vi "[FPGA] UART Demo.vi"() -> ()   [LabVIEW 2013]
uses:
  <vilib>/rvi/Emulation/niFpgaSctlEmulationGetInTimedLoop.vi
  <vilib>/rvi/Emulation/niFpgaEmulationReportErrorSimple.vi
  <vilib>/rvi/Emulation/niFpgaGetClockAttributes.vi
  <vilib>/rvi/Emulation/niFpgaCriticalErrorInLSC.vi
  UART 8N1/UART 8N1 (FPGA).lvlib
panel:
  in  "Write":bool
  in  "Write Data":u8
  in  "stop":bool
  out "Read Data":u8
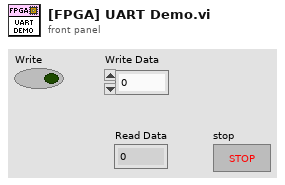
[diagram p1: front panel]
types:
  T1 = typedef "UART 8N1 (FPGA).lvlib/UART Ref.ctl" = cluster{"FPGA I/O":refnum<k21>, "Buffer Ref":refnum<k21>, "Stop Ref":refnum<k21>}
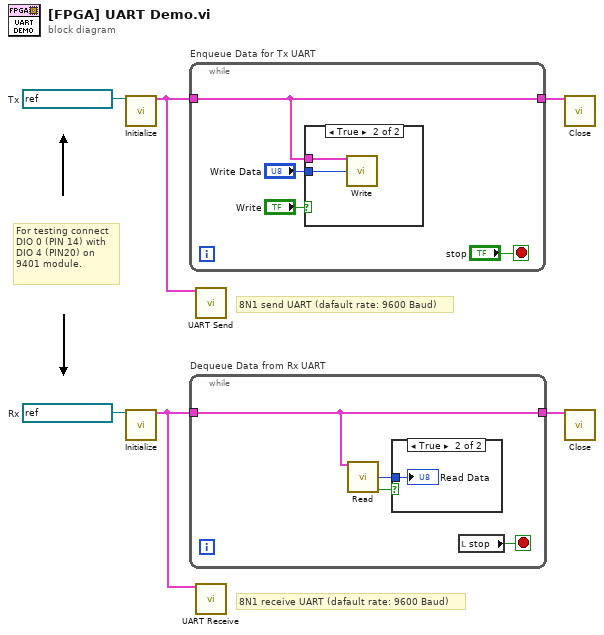
[diagram p0: block diagram]
diagram:
  w3 = refnum<k21> "Mod1/DIO0"  # Tx
  w6 = refnum<k21> "Mod1/DIO4"  # Rx
  # "For testing connect\nDIO 0 (PIN 14) with\nDIO 4 (PIN20) on \n9401 module."
  # "8N1 receive UART (dafault rate: 9600 Baud)"
  # "8N1 send UART (dafault rate: 9600 Baud)"
  n1 = call "Initialize.vi"("FPGA I/O"=w3) -> ("BPT Ref"=w2:T1)  [unwired: 14 in]
  n2 = call "Initialize.vi"("FPGA I/O"=w6) -> ("BPT Ref"=w4:T1)  [unwired: 14 in]
  n3 = while "Enqueue Data for Tx UART" {
    tunnel: w2 -> [w7]
    tunnel: [w7] -> w1
    stop <- "stop" stop-if-true
    n4 = case "Write" shown="True" "Write" {
      tunnel: w7 -> [_ w12]
      tunnel: "Write Data" -> [_ w11]
      frame False {
      }
      frame True {
        n5 = call "Write.vi"("UART Ref In"=w12, "Data"=w11) -> ()  [unwired: 12 in, 2 out]
      }
    }
  }
  n6 = while "Dequeue Data from Rx UART" {
    tunnel: [w15] -> w5
    tunnel: w4 -> [w15]
    stop <- w16 stop-if-true
    n7 = call "Read.vi"("UART Ref In"=w15) -> ("Data"=w14:u8, "Timed Out?"=w13:bool)  [unwired: 12 in, 1 out]
    n8 = case shown="True" w13 {
      tunnel: w14 -> [_ w17]
      frame False {
      }
      frame True {
        "Read Data" <- w17
      }
    }
    n9 = local read "stop"() -> (w16:bool)
  }
  n10 = call "UART Send.vi"("UART Ref In"=w2) -> ()  [unwired: 15 in]
  n11 = call "UART Receive.vi"("UART Ref"=w4) -> ()  [unwired: 15 in]
  n12 = call "Close.vi"("UART Ref"=w1) -> ()  [unwired: 15 in]
  n13 = call "Close.vi"("UART Ref"=w5) -> ()  [unwired: 15 in]
